vi "libssh2_sftp_close_handle.vi"(8 "error in (no error)":errorcluster, 11 "sftp handle":T1) -> (0 "error out":errorcluster)   [LabVIEW 2013, in "libssh2.lvlib"]
doc: "Close file handle."
uses:
  libssh2.lvlib
  SFTP Handle Refnum.ctl
  Global Settings.vi
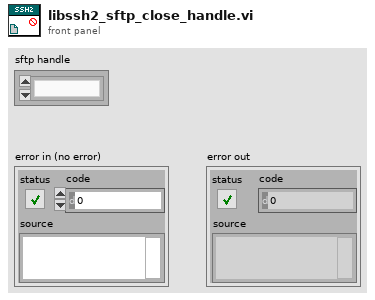
[diagram p1: front panel]
types:
  T1 = typedef "libssh2.lvlib/SFTP Handle Refnum.ctl" = refnum<k1>
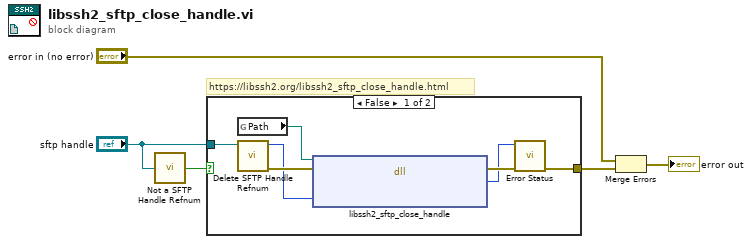
[diagram p0: block diagram]
diagram:
  # "https://libssh2.org/libssh2_sftp_close_handle.html"
  n1 = call "Not a SFTP Handle Refnum.vi"("sftp handle"="sftp handle") -> ("Not a SFTP Handle Refnum?"=w5:bool)
  n2 = case shown="False" w5 {
    tunnel: "sftp handle" -> [w11 _]
    tunnel: [w7 _] -> w4
    frame False {
      n3 = global read "Global Settings.vi" "Path"() -> (w12:path)
      n4 = call "Delete SFTP Handle Refnum.vi"("sftp handle"=w11) -> ("error out"=w10:errorcluster, "LIBSSH2_SFTP_HANDLE*"=w9:u64)  [unwired: 9 in]
      n5 = dll-call lib="C:/Users/pasca/source/repos/libssh2-labview/libssh2/libssh2**.*" fn="libssh2_sftp_close_handle"(path in=w12, error in=w10, "handle"=w9) -> (error out=w8:errorcluster, "return value"=w6:i32)  [unwired: 2 in, 1 out]
      n6 = call "Error Status.vi"("error in (no error)"=w8, "return value"=w6) -> ("error out"=w7:errorcluster)  [unwired: 8 in, 1 out]
    }
    frame True {
    }
  }
  n7 = Merge Errors("error in (no error)", w4) -> (→"error out":errorcluster)
